vi "Read Settings.vi"(8 "error in (no error)":errorcluster, 10 "Channel":string, 11 "Agilent DSO-X 3032A in":refnum<class "Agilent DSO-X 3032A.lvclass">) -> (0 "error out":errorcluster, 2 "Settings":T1={"Dt"=0.002, "#samples"=10000, "t0"=0.0} {"Dt" format="%.2e"}, 3 "Agilent DSO-X 3032A out":refnum<class "Agilent DSO-X 3032A.lvclass">)   [LabVIEW 2014, in "Agilent DSO-X 3032A.lvclass"]
uses:
  Agilent DSO-X 3032A.lvclass
  Channel Settings.ctl
  Agilent DSO-X 3032A.lvclass/Agilent DSO-X 3032A.ctl
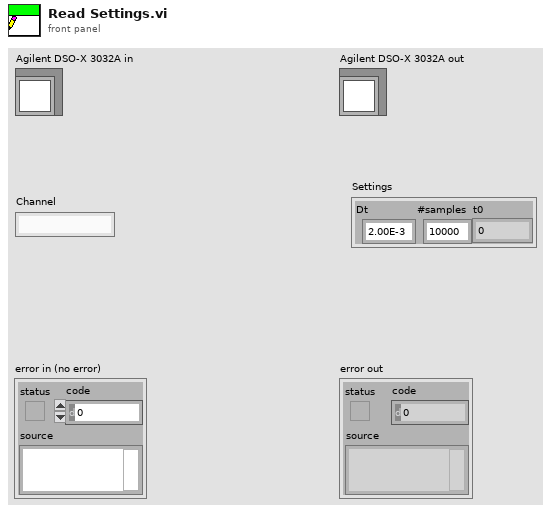
[diagram p1: front panel]
types:
  T1 = typedef "Agilent DSO-X 3032A.lvclass/Channel Settings.ctl" = cluster{"Dt":dbl, "#samples":i32, "t0":dbl}
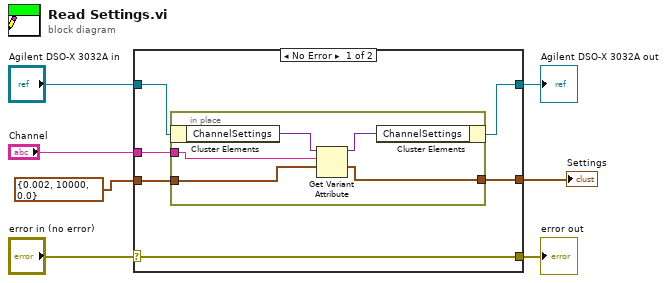
[diagram p0: block diagram]
diagram:
  n1 = case shown="No Error" "error in (no error)" {
    selector: "error in (no error)" -> [w13 w20]
    tunnel: [w13 w20] -> w6
    tunnel: [w11 w21] -> w4
    tunnel: "Agilent DSO-X 3032A in" -> [w12 w21]
    tunnel: "Channel" -> [w10 _]
    tunnel: [w9 w19] -> w2
    tunnel: T1 {"Dt"=0.002, "#samples"=10000, "t0"=0.0} ("Settings") -> [w8 w19]
    frame No Error {
      n2 = in-place {
        in-place-border: w10 -> [w16]
        in-place-border: [w15] -> w9
        in-place-border: w8 -> [w14]
        n3 = in-place-cluster #1(w12) -> ("ChannelSettings"=w18:variant)
        n4 = Get Variant Attribute(Variant=w18, name=w16, default value (empty Variant)=w14) -> (duplicate Variant=w17:variant, value=w15:T1)  [unwired: 1 in, 2 out]
        n5 = in-place-cluster #1("ChannelSettings"=w17) -> (w11:refnum<class "Agilent DSO-X 3032A.lvclass">)
      }
    }
    frame Error {
    }
  }
  "error out" <- w6
  "Agilent DSO-X 3032A out" <- w4
  "Settings" <- w2
